vi "Auto read numbers XYZ with camera.vi"() -> ()   [LabVIEW 2016]
uses:
  Classes/Controllers/Camera/Copy of Camera Folder/Machine Vision.ctl
  Classes/Controllers/Motion/Copy of A3200 Folder/A3200.lvclass
  D:/INTT/V1/Classes/Controllers/Motion/Copy of Motion Folder/Motion.lvclass
  <vilib>/Utility/file.llb/Read Delimited Spreadsheet (DBL).vi
  Classes/Controllers/Motion/Copy of Motion Folder/Motion.lvclass
  Classes/Controllers/Camera/Copy of Camera Folder/Camera.lvclass
panel:
  out "XYZTheta Out":dbl[](array[numeric])
  in  "stop":bool
  in  "start":bool
  out "XYZTheta Out 2":dbl[](array[numeric])
  in  "file path":path
  out "first row":dbl[](array[numeric])
  out "all rows":dbl[][](array[numeric])
  in  "Machine Vision":T1=enum."None"
  out "Camera":dbl[](array[numeric])
  in  "Stop":bool
  out "Image":T2(plugin-control)
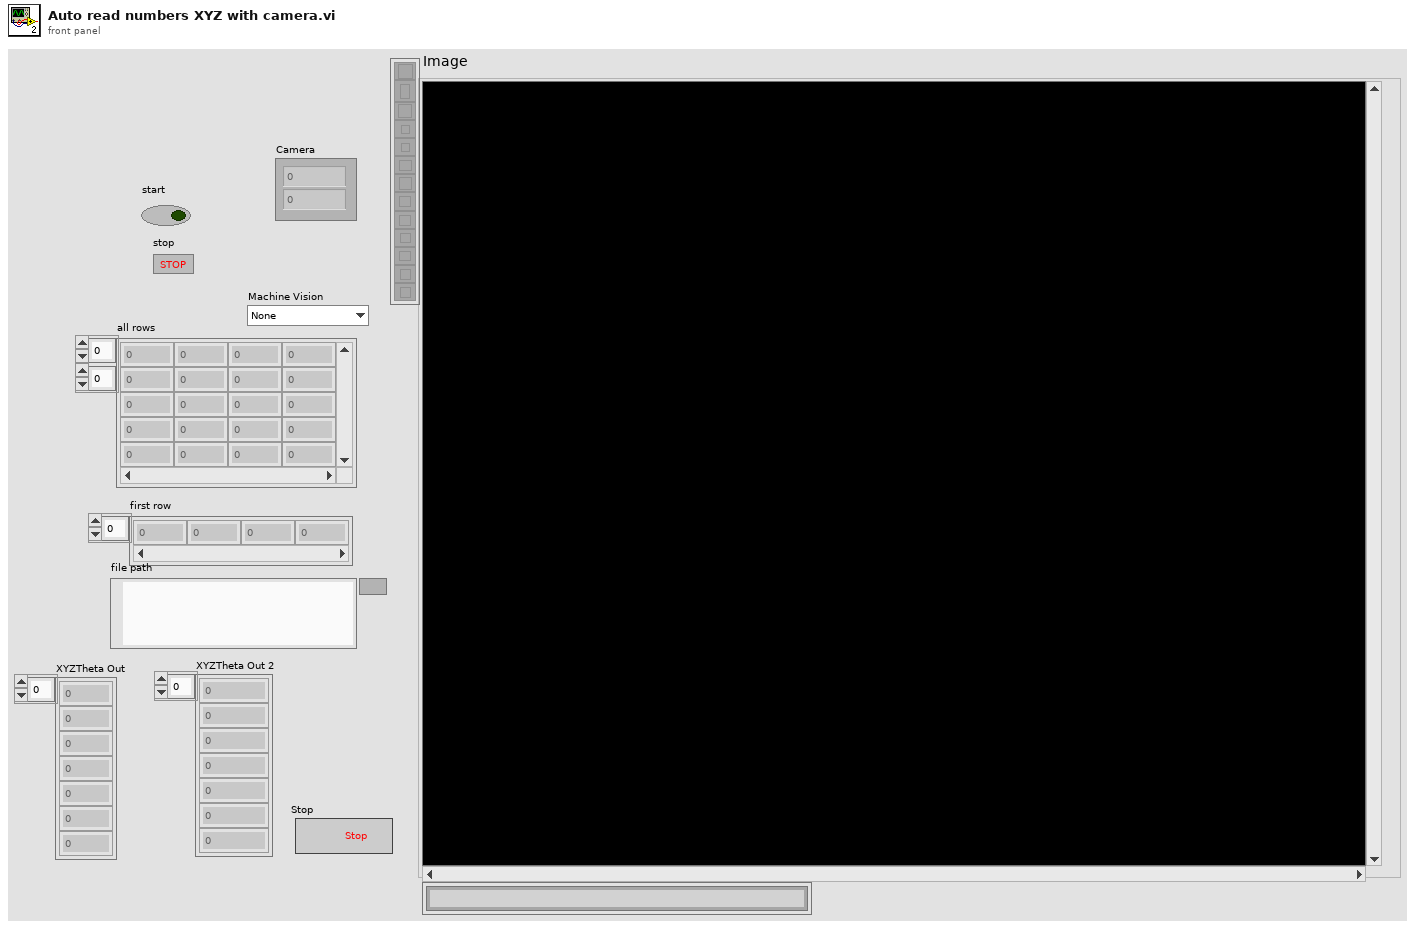
[diagram p1: front panel]
types:
  T1 = typedef "Camera.lvclass/Machine Vision.ctl" = enum16{"Focus", "LargeCircle", "None", "INTT HDI Mark", "INTT Sensor Cross", "INTT Chip Corner", "HPK Silicon", "circle"}
  T2 = typedef "IMAQ Image.ctl" = refnum<image>
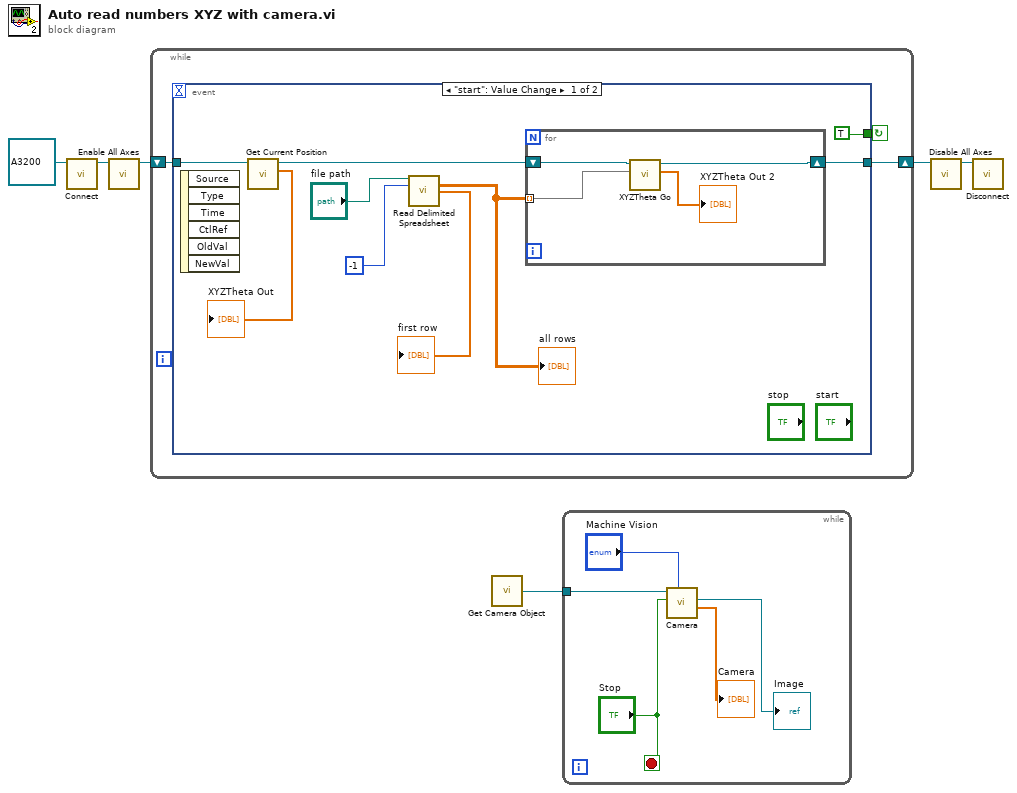
[diagram p0: block diagram]
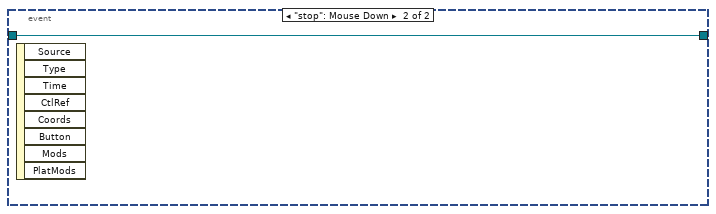
[diagram p2: hidden frame]
diagram:
  n1 = call-dynamic "Connect.vi"("Gantry in"=refnum<class "A3200.lvclass"> refnum ("Copy of A3200.lvclass")) -> ("Gantry out"=w4:refnum<class "A3200.lvclass">)  [unwired: 9 in, 1 out]
  n2 = call-dynamic "Enable All Axes.vi"("A3200 in"=w4) -> ("A3200 out"=w3:refnum<class "A3200.lvclass">)  [unwired: 9 in, 1 out]
  n3 = while {
    shift-right: [w9] -> w2
    shift-left: w3 -> [w8]
    stop <- w7 continue-if-true
    n4 = event shown="[0] \"start\": Value Change" {
      selector: _ -> [_ _]
      dyn-events: _ -> [_ _]
      timeout: _ -> [_ _]
      tunnel: [w18 w23] -> w9
      tunnel: w8 -> [w16 w23]
      tunnel: [TRUE _] -> w7
      event "start": Value Change {
        n5 = event-data() -> ()  [unwired: 1 in, 6 out]
        n6 = call-dynamic "Get Current Position.vi"("Gantry in"=w16) -> ("XYZTheta Out"=→"XYZTheta Out":dbl[], "Gantry out"=w15:refnum<class "A3200.lvclass">)  [unwired: 8 in, 1 out]
        n7 = call-poly <vilib>:"Read Delimited Spreadsheet.vi"("file path (dialog if empty)"="file path", "number of rows (all:-1)"=-1) -> ("all rows"=w10:dbl[][], "first row"=→"first row":dbl[])  [unwired: 8 in, 4 out]
        "all rows" <- w10
        n8 = for {
          shift-right: [w22] -> w18
          shift-left: w15 -> [w20]
          tunnel: w10 -> [w19] mode=indexing
          n9 = call "XYZTheta Go.vi"("XYZTheta In"=w19, "Motion in"=w20) -> ("XYZTheta Out"=→"XYZTheta Out 2":dbl[], "Motion out"=w22:refnum<class "A3200.lvclass">)  [unwired: 7 in, 1 out]
        }
      }
      event "stop": Mouse Down {
        n10 = event-data() -> ()  [unwired: 1 in, 8 out]
      }
    }
  }
  n11 = call "Get Camera Object.vi"() -> ("Camera out"=w6:refnum<class "Camera.lvclass">)  [unwired: 10 in, 1 out]
  n12 = while {
    tunnel: w6 -> [w27]
    stop <- "Stop" stop-if-true
    n13 = call "Camera.vi"("Machine Vision"="Machine Vision", "Stop"="Stop", "Camera in"=w27) -> ("Camera"=→"Camera":dbl[], "Image"=→"Image":T2)  [unwired: 3 in, 4 out]
  }
  n14 = call-dynamic "Disable All Axes.vi"("Gantry in"=w2) -> ("Gantry out"=w1:refnum<class "A3200.lvclass">)  [unwired: 9 in, 1 out]
  n15 = call-dynamic "Disconnect.vi"("Gantry in"=w1) -> ()  [unwired: 9 in, 1 out]
